vi "lab1Text.vi"() -> (3 "String":string)   [LabVIEW 2015]
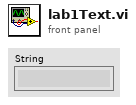
[diagram p1: front panel]
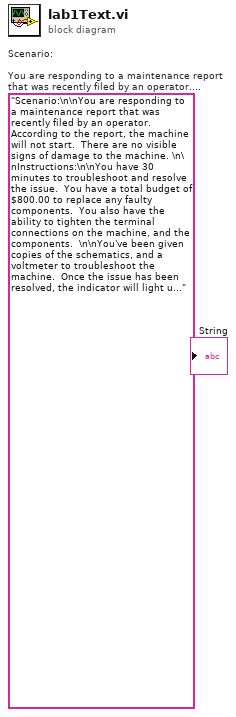
[diagram p0: block diagram]
diagram:
  w1 = "Scenario:\n\nYou are responding to a maintenance report that was recently filed by an operator.  According to the report, the machine will not start.  There are no visible signs of damage to the machine. \n\nInstructions:\n\nYou have 30 minutes to troubleshoot and resolve the issue.  You have a total budget of $800.00 to replace any faulty components.  You also have the ability to tighten the terminal connections on the machine, and the components.  \n\nYou've been given copies of the schematics, and a voltmeter to troubleshoot the machine.  Once the issue has been resolved, the indicator will light up.  It is recommended that you take some time to manually verify that the issue has been resolved.  When you are finished, be sure to click the 'Close Lab' button."  # Scenario:  You are responding to a maintenance report that was recently filed by an operator.  According to the report, the machine will not start.  There are no visible signs of damage to the machine.   Instructions:  You have 30 minutes to troubleshoot and resolve the issue.  You have a total budget of $800.00 to replace any faulty components.  You also have the ability to tighten the terminal connections on the machine, and the components.    You've been given copies of the schematics, and a voltmeter to troubleshoot the machine.  Once the issue has been resolved, the indicator will light up.  It is recommended that you take some time to manually verify that the issue has been resolved.  When you are finished, be sure to click the 'Close Lab' button.
  "String" <- w1
